vi "CTL Pump_Controller.vi"(6 "error in (no error)":errorcluster, 7 "Full Config":T1={"Bench Config"={"Name"="OLR001", {"Step Levels"=0.05, "Tolerance"=0.01, "Sample Rate"=0.05, "Resistor"=100.0, "M Level Cal"=1.0, "[B Level Cal"=0.0, "Max Fill Rate"=0.025, "Empty Inches"=10.0, "Full Inches"=10.0}}, "Test Value Table "=[[0.0, 0.0, 0.0, 0.0, 0.0, 0.0, 0.0, 0.0, 0.0, 0.0], [100.0, 2.0, 7.91, 8.01, 7.55, 7.65, 7.685, 7.785, 7.325, 7.425], [200.0, 3.0, 7.46, 7.56, 7.1, 7.2, 7.235, 7.335, 6.875, 6.975], [300.0, 4.0, 7.01, 7.11, 6.65, 6.75, 6.785, 6.885, 6.425, 6.525], [400.0, 5.0, 6.56, 6.66, 6.2, 6.3, 6.335, 6.435, 5.975, 6.075], [500.0, 6.0, 6.11, 6.21, 5.75, 5.85, 5.885, 5.985, 5.525, 5.625], [600.0, 7.0, 5.66, 5.76, 5.3, 5.4, 5.435, 5.535, 5.075, 5.175], [700.0, 8.0, 5.21, 5.31, 4.85, 4.95, 4.985, 5.085, 4.625, 4.725], [800.0, 9.0, 4.76, 4.86, 4.4, 4.5, 4.535, 4.635, 4.175, 4.275], [900.0, 10.0, 4.31, 4.41, 3.95, 4.05, 4.085, 4.185, 3.725, 3.825], [1000.0, 11.0, 3.86, 3.96, 3.5, 3.6, 3.635, 3.735, 3.275, 3.375], [1100.0, 12.0, 3.41, 3.51, 3.05, 3.15, 3.185, 3.285, 2.825, 2.925]], "Table Col Titles"=[["A Resist", "A Tolerence", "A Fill Lo", "A Fill Hi", "A Drain Lo", "A Drain Hi", "B Fill Lo", "B Fill Hi", "B Drain Lo", "B Drain Hi"]], "Pump CtlRef In"={"Fill "=refnum, "Drain"=refnum, "Level PV"=refnum, "Flow Rate%"=refnum, "Run Test"=refnum, "Sim"=refnum, "Jog"=refnum, "Level SP"=refnum}, "Bench Status"={"Pump Status"=refnum, "Instrumnet\n Status"=refnum}}, 9 "Level PV":dbl=0.024999999999999842, 10 "Level SP":dbl, 11 "TEST State In":T5(ring)=enum."Done") -> (0 "TEST State Out":T5(ring)=enum."Done", 1 "Drain Out":bool, 2 "Fill Out":bool, 4 "error out":errorcluster)   [LabVIEW 2024]
doc: "Simulates the level inch (0 = empty) and Level Sense (8.5 = empty).\nIf Test Status is manual then the Drain and Fill buttons cause the level to decrese or increase.\nOtherwise, drain and fill are determnied by the state variable and the difference between Level SP (Set Point) and Level PV (Present Value)\nThe level rate of change is determined by the Flow Rate setting."
uses:
  Control Definitions/Def FullCfg.ctl
  Control Definitions/Def BenchCfg.ctl
  Control Definitions/Def PumpCtlRefs.ctl
  Control Definitions/Def Bench Status.ctl
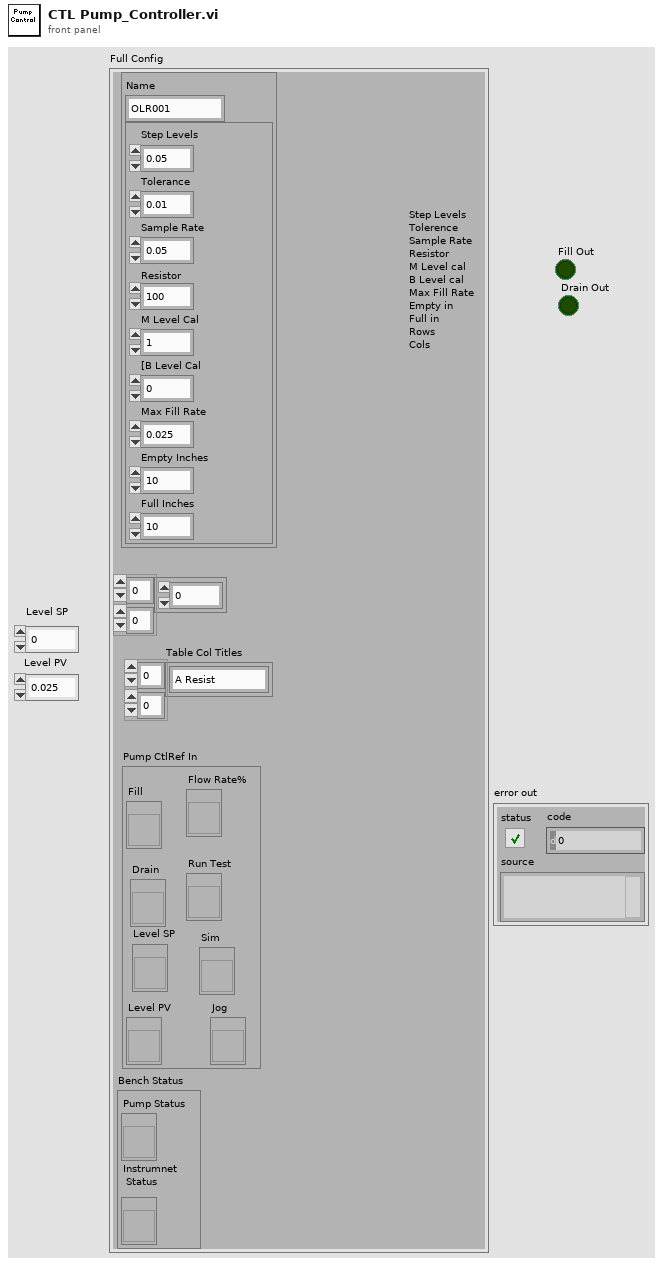
[diagram p1: front panel]
types:
  T1 = typedef "Def FullCfg.ctl" = cluster{"Bench Config":T2, "Test Value Table ":dbl[][], "Table Col Titles":string[][], "Pump CtlRef In":T3, "Bench Status":T4}
  T2 = typedef "Def BenchCfg.ctl" = cluster{"Name":string, cluster{"Step Levels":dbl, "Tolerance":dbl, "Sample Rate":dbl, "Resistor":dbl, "M Level Cal":dbl, "[B Level Cal":dbl, "Max Fill Rate":dbl, "Empty Inches":dbl, "Full Inches":dbl}}
  T3 = typedef "Def PumpCtlRefs.ctl" = cluster{"Fill ":refnum<vi>, "Drain":refnum<vi>, "Level PV":refnum<vi>, "Flow Rate%":refnum<vi>, "Run Test":refnum<vi>, "Sim":refnum<vi>, "Jog":refnum<vi>, "Level SP":refnum<vi>}
  T4 = typedef "Def Bench Status.ctl" = cluster{"Pump Status":refnum<vi>, "Instrumnet\n Status":refnum<vi>}
  T5 = enum16{"MANUAL", "Start", "Filling", "FULL", "Draining", "EMPTY", "Done"}
  T6 = cluster{"Step Levels":dbl, "Tolerance":dbl, "Sample Rate":dbl, "Resistor":dbl, "M Level Cal":dbl, "[B Level Cal":dbl, "Max Fill Rate":dbl, "Empty Inches":dbl, "Full Inches":dbl}
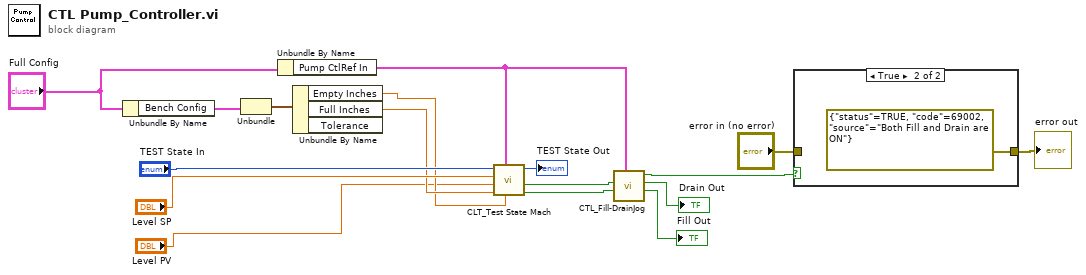
[diagram p0: block diagram]
diagram:
  n1 = Unbundle By Name("Full Config") -> ("Bench Config"=w12:T2)
  n2 = Unbundle(w12) -> (w11:T6)  [unwired: 1 out]
  n3 = Unbundle By Name("Full Config") -> ("Pump CtlRef In"=w6:T3)
  n4 = Unbundle By Name(w11) -> ("Empty Inches"=w8:dbl, "Full Inches"=w10:dbl)  [unwired: 1 out]
  n5 = call "CLT_Test State Mach.vi"("Empty in"=w8, "Pump CtlRef In"=w6, "Full in"=w10, "Level PV"="Level PV", "Level SP"="Level SP", "TEST STATUS In"="TEST State In") -> ("Fill Cmd"=w1:bool, "Drain Cmd"=w2:bool, "TEST STATUS Out"=→"TEST State Out":T5)  [unwired: 2 in, 1 out]
  n6 = call "CTL_Fill-DrainJog.vi"("Pump CtlRef In"=w6, "Fill Cmd"=w1, "Drain Cmd"=w2) -> ("Fill Out"=→"Fill Out":bool, "Drain Out"=→"Drain Out":bool, "Err"=w5:bool)  [unwired: 4 in, 2 out]
  n7 = case shown="True" w5 {
    tunnel: "error in (no error)" -> [w18 _]
    tunnel: [w18 errorcluster {"status"=TRUE, "code"=69002, "source"="Both Fill and Drain are ON"} ("error in (no error)")] -> w16
    frame False {
    }
    frame True {
    }
  }
  "error out" <- w16
